vi "SplitTileCode.vi"() -> ()   [LabVIEW 2019, in "RT_Game.lvlib" / "Engine.lvclass"]
uses:
  Engine.lvclass
panel:
  in  "Rotation":enum16{"None", "Right", "Down", "Left"}(ring)
  in  "color_to_replace":fxp<+,3,3>
  in  "replacecolor":fxp<+,3,3>
  in  "Flip":enum16{"None", "LeftRight", "UpDown", "Both"}(ring)
  in  "color_to_replace 2":fxp<+,3,3>
  in  "replacecolor 2":fxp<+,3,3>
  out "TileCode":u32
  in  "Tilenumber":u16
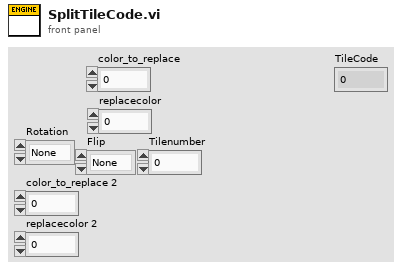
[diagram p1: front panel]
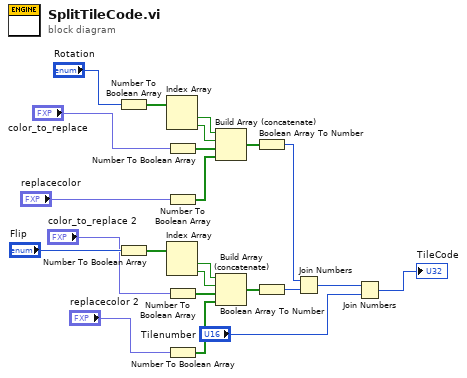
[diagram p0: block diagram]
diagram:
  n1 = Number To Boolean Array(number="Rotation") -> (Boolean array=w10:bool[])
  n2 = Number To Boolean Array(number="Flip") -> (Boolean array=w18:bool[])
  n3 = Index Array(array=w10) -> (element #1=w11:bool, element #2=w12:bool)  [unwired: 2 in]
  n4 = Index Array(array=w18) -> (element #1=w17:bool, element #2=w16:bool)  [unwired: 2 in]
  n5 = Number To Boolean Array(number="color_to_replace") -> (Boolean array=w13:bool[])
  n6 = Number To Boolean Array(number="replacecolor") -> (Boolean array=w9:bool[])
  n7 = Number To Boolean Array(number="color_to_replace 2") -> (Boolean array=w15:bool[])
  n8 = Number To Boolean Array(number="replacecolor 2") -> (Boolean array=w8:bool[])
  n9 = Build Array (concatenate)(w11, w12, w13, w9) -> (w14:bool[])
  n10 = Build Array (concatenate)(w17, w16, w15, w8) -> (w19:bool[])
  n11 = Boolean Array To Number(Boolean array=w14) -> (number=w21:u8)
  n12 = Boolean Array To Number(Boolean array=w19) -> (number=w22:u8)
  n13 = Join Numbers(hi=w21, lo=w22) -> ((hi.lo)=w20:u16)
  n14 = Join Numbers(hi=w20, lo="Tilenumber") -> ((hi.lo)=→"TileCode":u32)
